vi "p70MonInv.vi"() -> ()   [LabVIEW 2013]
panel:
  out "division":dbl[](array[numeric])
  out "Array 4":dbl[](array[numeric])
  out "Patrones":dbl[][](array[numeric])
  out "Array 2":dbl[][](array[numeric])
  out "Array":dbl[][](array[numeric])
  out "appended array":dbl[](array[numeric])
  out "new picture 2":picture
  out "new picture":picture
  in  "path to BMP file":path
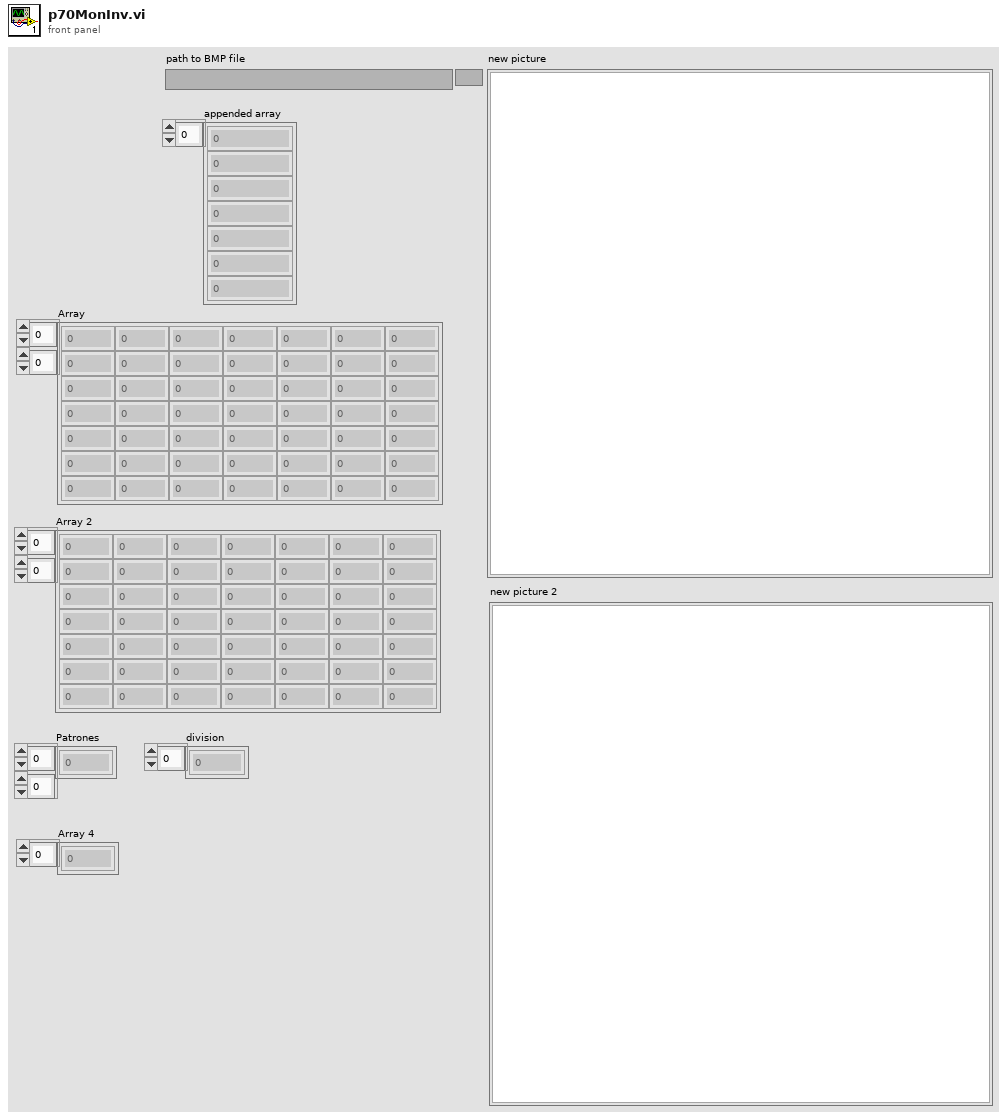
[diagram p1: front panel]
types:
  T1 = typedef "imagedata.ctl" = cluster{"image type":i32, "image depth":i32, "image":u8[], "mask":u8[], "colors":u32[], "Rectangle":cluster{"left":i16, "top":i16, "right":i16, "bottom":i16}}
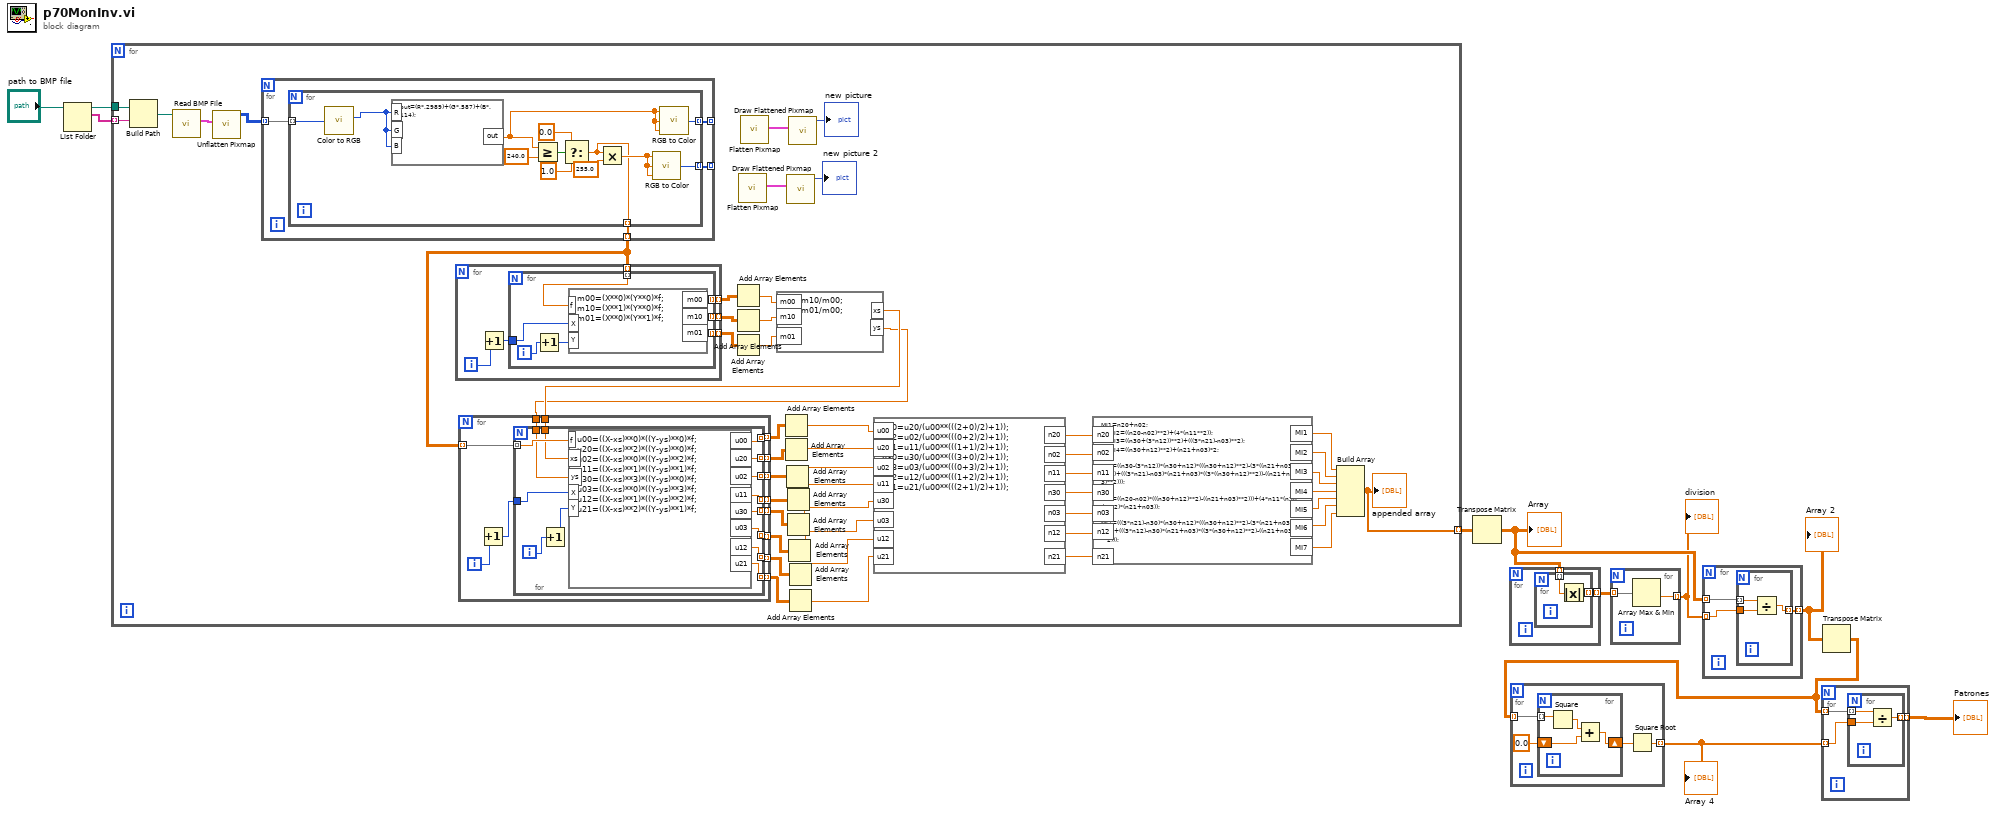
[diagram p0: block diagram]
diagram:
  n1 = List Folder(path="path to BMP file") -> (path out=w9:path, filenames=w10:string[])  [unwired: 3 in, 2 out]
  n2 = for {
    tunnel: w10 -> [w15] mode=indexing
    tunnel: w9 -> [w14]
    tunnel: [w12] -> w5 mode=indexing
    n3 = Build Path(base path=w14, name or relative path=w15) -> (appended path=w13:path)
    n4 = call <vilib>:"Read BMP File.vi"("path to BMP file"=w13) -> ("image data"=w17:T1)  [unwired: 8 in, 2 out]
    n5 = call <vilib>:"Unflatten Pixmap.vi"("image data"=w17) -> ("24-bit pixmap"=w16:u32[][])  [unwired: 4 in, 6 out]
    n6 = for {
      tunnel: w16 -> [w104] mode=indexing
      tunnel: [w103] -> _ mode=indexing
      tunnel: [w102] -> _ mode=indexing
      tunnel: [w101] -> w50 mode=indexing
      n7 = for {
        tunnel: w104 -> [w116] mode=indexing
        tunnel: [w115] -> w103 mode=indexing
        tunnel: [w106] -> w102 mode=indexing
        tunnel: [w105] -> w101 mode=indexing
        n8 = call <vilib>:"Color to RGB.vi"("Color"=w116) -> ("R"=w114:u8)  [unwired: 3 out]
        n9 = formula code="out=(R*.2989)+(G*.587)+(B*.114);"("R"=w114, "G"=w114, "B"=w114) -> ("out"=w112:dbl)
        n10 = Greater Or Equal?(x=w112, y=240.0) -> (x >= y?=w113:bool)
        n11 = Select(t=0.0, s=w113, f=1.0) -> (s? t:f=w105:dbl)
        n12 = Multiply(x=w105, y=255.0) -> (x*y=w107:dbl)
        n13 = call <vilib>:"RGB to Color.vi"("B"=w107, "G"=w107, "R"=w107) -> ("Color"=w106:u32)
        n14 = call <vilib>:"RGB to Color.vi"("B"=w112, "G"=w112, "R"=w112) -> ("Color"=w115:u32)
      }
    }
    n15 = for {
      tunnel: w50 -> [w92] mode=indexing
      tunnel: [w90] -> w56 mode=indexing
      tunnel: [w89] -> w55 mode=indexing
      tunnel: [w88] -> w54 mode=indexing
      i -> [w93]
      n16 = Increment(x=w93) -> (x+1=w91:i32)
      n17 = for {
        tunnel: w92 -> [w100] mode=indexing
        tunnel: w91 -> [w99]
        tunnel: [w96] -> w90 mode=indexing
        tunnel: [w95] -> w89 mode=indexing
        tunnel: [w94] -> w88 mode=indexing
        i -> [w98]
        n18 = Increment(x=w98) -> (x+1=w97:i32)
        n19 = formula code="m00=(X**0)*(Y**0)*f;\nm10=(X**1)*(Y**0)*f;\nm01=(X**0)*(Y**1)*f;"("X"=w99, "Y"=w97, "f"=w100) -> ("m00"=w96:dbl, "m10"=w95:dbl, "m01"=w94:dbl)
      }
    }
    n20 = Add Array Elements(numeric array=w56) -> (sum=w53:dbl)
    n21 = Add Array Elements(numeric array=w55) -> (sum=w52:dbl)
    n22 = Add Array Elements(numeric array=w54) -> (sum=w51:dbl)
    n23 = call <vilib>:"Flatten Pixmap.vi"() -> ("image data"=w57:T1)  [unwired: 11 in]
    n24 = call <vilib>:"Flatten Pixmap.vi"() -> ("image data"=w60:T1)  [unwired: 11 in]
    n25 = formula code="xs=m10/m00;\nys=m01/m00;"("m00"=w53, "m10"=w52, "m01"=w51) -> ("xs"=w49:dbl, "ys"=w48:dbl)
    n26 = for {
      tunnel: w50 -> [w73] mode=indexing
      tunnel: w49 -> [w72]
      tunnel: w48 -> [w71]
      tunnel: [w68] -> w47 mode=indexing
      tunnel: [w67] -> w46 mode=indexing
      tunnel: [w66] -> w45 mode=indexing
      tunnel: [w65] -> w44 mode=indexing
      tunnel: [w64] -> w43 mode=indexing
      tunnel: [w63] -> w42 mode=indexing
      tunnel: [w62] -> w41 mode=indexing
      tunnel: [w61] -> w40 mode=indexing
      i -> [w70]
      n27 = Increment(x=w70) -> (x+1=w69:i32)
      n28 = for {
        tunnel: w73 -> [w87] mode=indexing
        tunnel: w72 -> [w86]
        tunnel: w71 -> [w85]
        tunnel: w69 -> [w84]
        tunnel: [w81] -> w68 mode=indexing
        tunnel: [w80] -> w67 mode=indexing
        tunnel: [w79] -> w66 mode=indexing
        tunnel: [w78] -> w65 mode=indexing
        tunnel: [w77] -> w64 mode=indexing
        tunnel: [w76] -> w63 mode=indexing
        tunnel: [w75] -> w62 mode=indexing
        tunnel: [w74] -> w61 mode=indexing
        i -> [w83]
        n29 = Increment(x=w83) -> (x+1=w82:i32)
        n30 = formula code="u00=((X-xs)**0)*((Y-ys)**0)*f;\nu20=((X-xs)**2)*((Y-ys)**0)*f;\nu02=((X-xs)**0)*((Y-ys)**2)*f;\nu11=((X-xs)**1)*((Y-ys)**1)*f;\nu30=((X-xs)**3)*((Y-ys)**0)*f;\nu03=((X-xs)**0)*((Y-ys)**3)*f;\nu12=((X-xs)**1)*((Y-ys)**2)*f;\nu21=((X-xs)**2)*((Y-ys)**1)*f;"("f"=w87, "xs"=w86, "ys"=w85, "X"=w84, "Y"=w82) -> ("u00"=w81:dbl, "u20"=w80:dbl, "u02"=w79:dbl, "u11"=w78:dbl, "u30"=w77:dbl, "u03"=w76:dbl, "u12"=w75:dbl, "u21"=w74:dbl)
      }
    }
    n31 = Add Array Elements(numeric array=w47) -> (sum=w39:dbl)
    n32 = Add Array Elements(numeric array=w46) -> (sum=w38:dbl)
    n33 = Add Array Elements(numeric array=w45) -> (sum=w37:dbl)
    n34 = Add Array Elements(numeric array=w44) -> (sum=w36:dbl)
    n35 = Add Array Elements(numeric array=w43) -> (sum=w35:dbl)
    n36 = Add Array Elements(numeric array=w42) -> (sum=w34:dbl)
    n37 = Add Array Elements(numeric array=w41) -> (sum=w33:dbl)
    n38 = Add Array Elements(numeric array=w40) -> (sum=w32:dbl)
    n39 = call <vilib>:"Draw Flattened Pixmap.vi"("image data"=w57) -> ("new picture"=→"new picture 2":picture)  [unwired: 8 in]
    n40 = call <vilib>:"Draw Flattened Pixmap.vi"("image data"=w60) -> ("new picture"=→"new picture":picture)  [unwired: 8 in]
    n41 = formula code="n20=u20/(u00**(((2+0)/2)+1));\nn02=u02/(u00**(((0+2)/2)+1));\nn11=u11/(u00**(((1+1)/2)+1));\nn30=u30/(u00**(((3+0)/2)+1));\nn03=u03/(u00**(((0+3)/2)+1));\nn12=u12/(u00**(((1+2)/2)+1));\nn21=u21/(u00**(((2+1)/2)+1));"("u00"=w39, "u20"=w38, "u02"=w37, "u11"=w36, "u30"=w35, "u03"=w34, "u12"=w33, "u21"=w32) -> ("n20"=w31:dbl, "n02"=w30:dbl, "n11"=w29:dbl, "n30"=w28:dbl, "n03"=w27:dbl, "n12"=w26:dbl, "n21"=w25:dbl)
    n42 = formula code="MI1=n20+n02;\n    MI2=((n20-n02)**2)+(4*(n11**2));\n    MI3=((n30+(3*n12))**2)+(((3*n21)-n03)**2);\n    MI4=((n30+n12)**2)+(n21+n03)*2;\n    MI5=((n30-(3*n12))*(n30+n12)*(((n30+n12)**2)-(3*((n21+n03)**2))))+(((3*n21)-n03)*(n21+n03)*((3*((n30+n12)**2))-((n21+n03)**2)));\n    MI6=((n20-n02)*(((n30+n12)**2)-((n21+n03)**2)))+(4*n11*(n30+n12)*(n21+n03));\n    MI7=(((3*n21)-n30)*(n30+n12)*(((n30+n12)**2)-(3*(n21+n03)**2)))+(((3*n12)-n30)*(n21+n03)*((3*(n30+n12)**2)-((n21+n03)**2)));"("n20"=w31, "n02"=w30, "n11"=w29, "n30"=w28, "n03"=w27, "n12"=w26, "n21"=w25) -> ("MI1"=w24:dbl, "MI2"=w23:dbl, "MI3"=w22:dbl, "MI4"=w21:dbl, "MI5"=w20:dbl, "MI6"=w19:dbl, "MI7"=w18:dbl)
    n43 = Build Array(w24, w23, w22, w21, w20, w19, w18) -> (w12:dbl[])
    "appended array" <- w12
  }
  n44 = Transpose Matrix(1:w5) -> (0:w7:dbl[][])
  "Array" <- w7
  n45 = for {
    tunnel: w7 -> [w118] mode=indexing
    tunnel: [w117] -> w8 mode=indexing
    n46 = for {
      tunnel: w118 -> [w120] mode=indexing
      tunnel: [w119] -> w117 mode=indexing
      n47 = Absolute Value(x=w120) -> (abs(x)=w119:dbl)
    }
  }
  n48 = for {
    tunnel: w8 -> [w122] mode=indexing
    tunnel: [w121] -> w6 mode=indexing
    n49 = Array Max & Min(array=w122) -> (min value=w121:dbl)  [unwired: 3 out]
  }
  "division" <- w6
  n50 = for {
    tunnel: w7 -> [w125] mode=indexing
    tunnel: w6 -> [w124] mode=indexing
    tunnel: [w123] -> w2 mode=indexing
    n51 = for {
      tunnel: w125 -> [w127] mode=indexing
      tunnel: w124 -> [w128]
      tunnel: [w126] -> w123 mode=indexing
      n52 = Divide(x=w127, y=w128) -> (x/y=w126:dbl)
    }
  }
  "Array 2" <- w2
  n53 = Transpose Matrix(1:w2) -> (0:w1:dbl[][])
  n54 = for {
    tunnel: w1 -> [w132] mode=indexing
    tunnel: [w129] -> w4 mode=indexing
    n55 = for {
      tunnel: w132 -> [w136] mode=indexing
      shift-right: [w133] -> w130
      shift-left: 0.0 -> [w134]
      n56 = Square(x=w136) -> (x^2=w135:dbl)
      n57 = Add(x=w135, y=w134) -> (x+y=w133:dbl)
    }
    n58 = Square Root(x=w130) -> (sqrt(x)=w129:dbl)
  }
  "Array 4" <- w4
  n59 = for {
    tunnel: w1 -> [w139] mode=indexing
    tunnel: w4 -> [w138] mode=indexing
    tunnel: [w137] -> w3 mode=indexing
    n60 = for {
      tunnel: w139 -> [w142] mode=indexing
      tunnel: w138 -> [w141]
      tunnel: [w140] -> w137 mode=indexing
      n61 = Divide(x=w142, y=w141) -> (x/y=w140:dbl)
    }
  }
  "Patrones" <- w3
